vi "Write Container.vi"(10 "Sample Transfer Container":T1, 11 "Read Sample from Container Msg in":refnum<class "Read Sample from Container Msg.lvclass">) -> (3 "Read Sample from Container Msg out":refnum<class "Read Sample from Container Msg.lvclass">)   [LabVIEW 2015, in "cRIO-Carbondioxide.lvlib" / "CO2-Actor.lvlib" / "Read Sample from Container Msg.lvclass"]
uses:
  Read Sample from Container Msg.lvclass
  Controls/Sample Transfer Container Enumerator.ctl
  Read Sample from Container Msg.lvclass/Read Sample from Container Msg.ctl
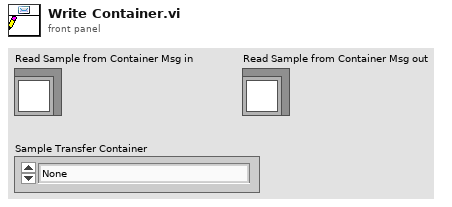
[diagram p1: front panel]
types:
  T1 = typedef "Sample Transfer Container Enumerator.ctl" = enum16{"None", "Sample 1", "Sample 2", "Sample 3", "Sample 4", "Sample 5", "Storage 01", "Storage 02", "Storage 03", "Storage 04", "Storage 05", "Storage 06", "Storage 07", "Storage 08", "Storage 09", "Storage 10", "Storage 11", "Storage 12", "Syringe", "Undefined"}
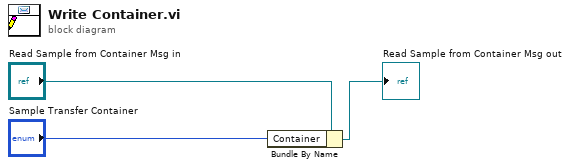
[diagram p0: block diagram]
diagram:
  n1 = Bundle By Name(cluster="Read Sample from Container Msg in", "Container"="Sample Transfer Container") -> (→"Read Sample from Container Msg out":refnum<class "Read Sample from Container Msg.lvclass">)
